vi "TestItemsIndex.vi"(6 "TestItemIndexIn":i32, 8 "ErrorIn":errorcluster, 9 "GuiRef":T1, 11 "Fail项目":string[](array[string])) -> (0 "ErrorOut":errorcluster, 1 "GuiRefOut":T1)   [LabVIEW 2013]
uses:
  GlobValue.vi
panel:
  out "Item Names":string[][](array[string])
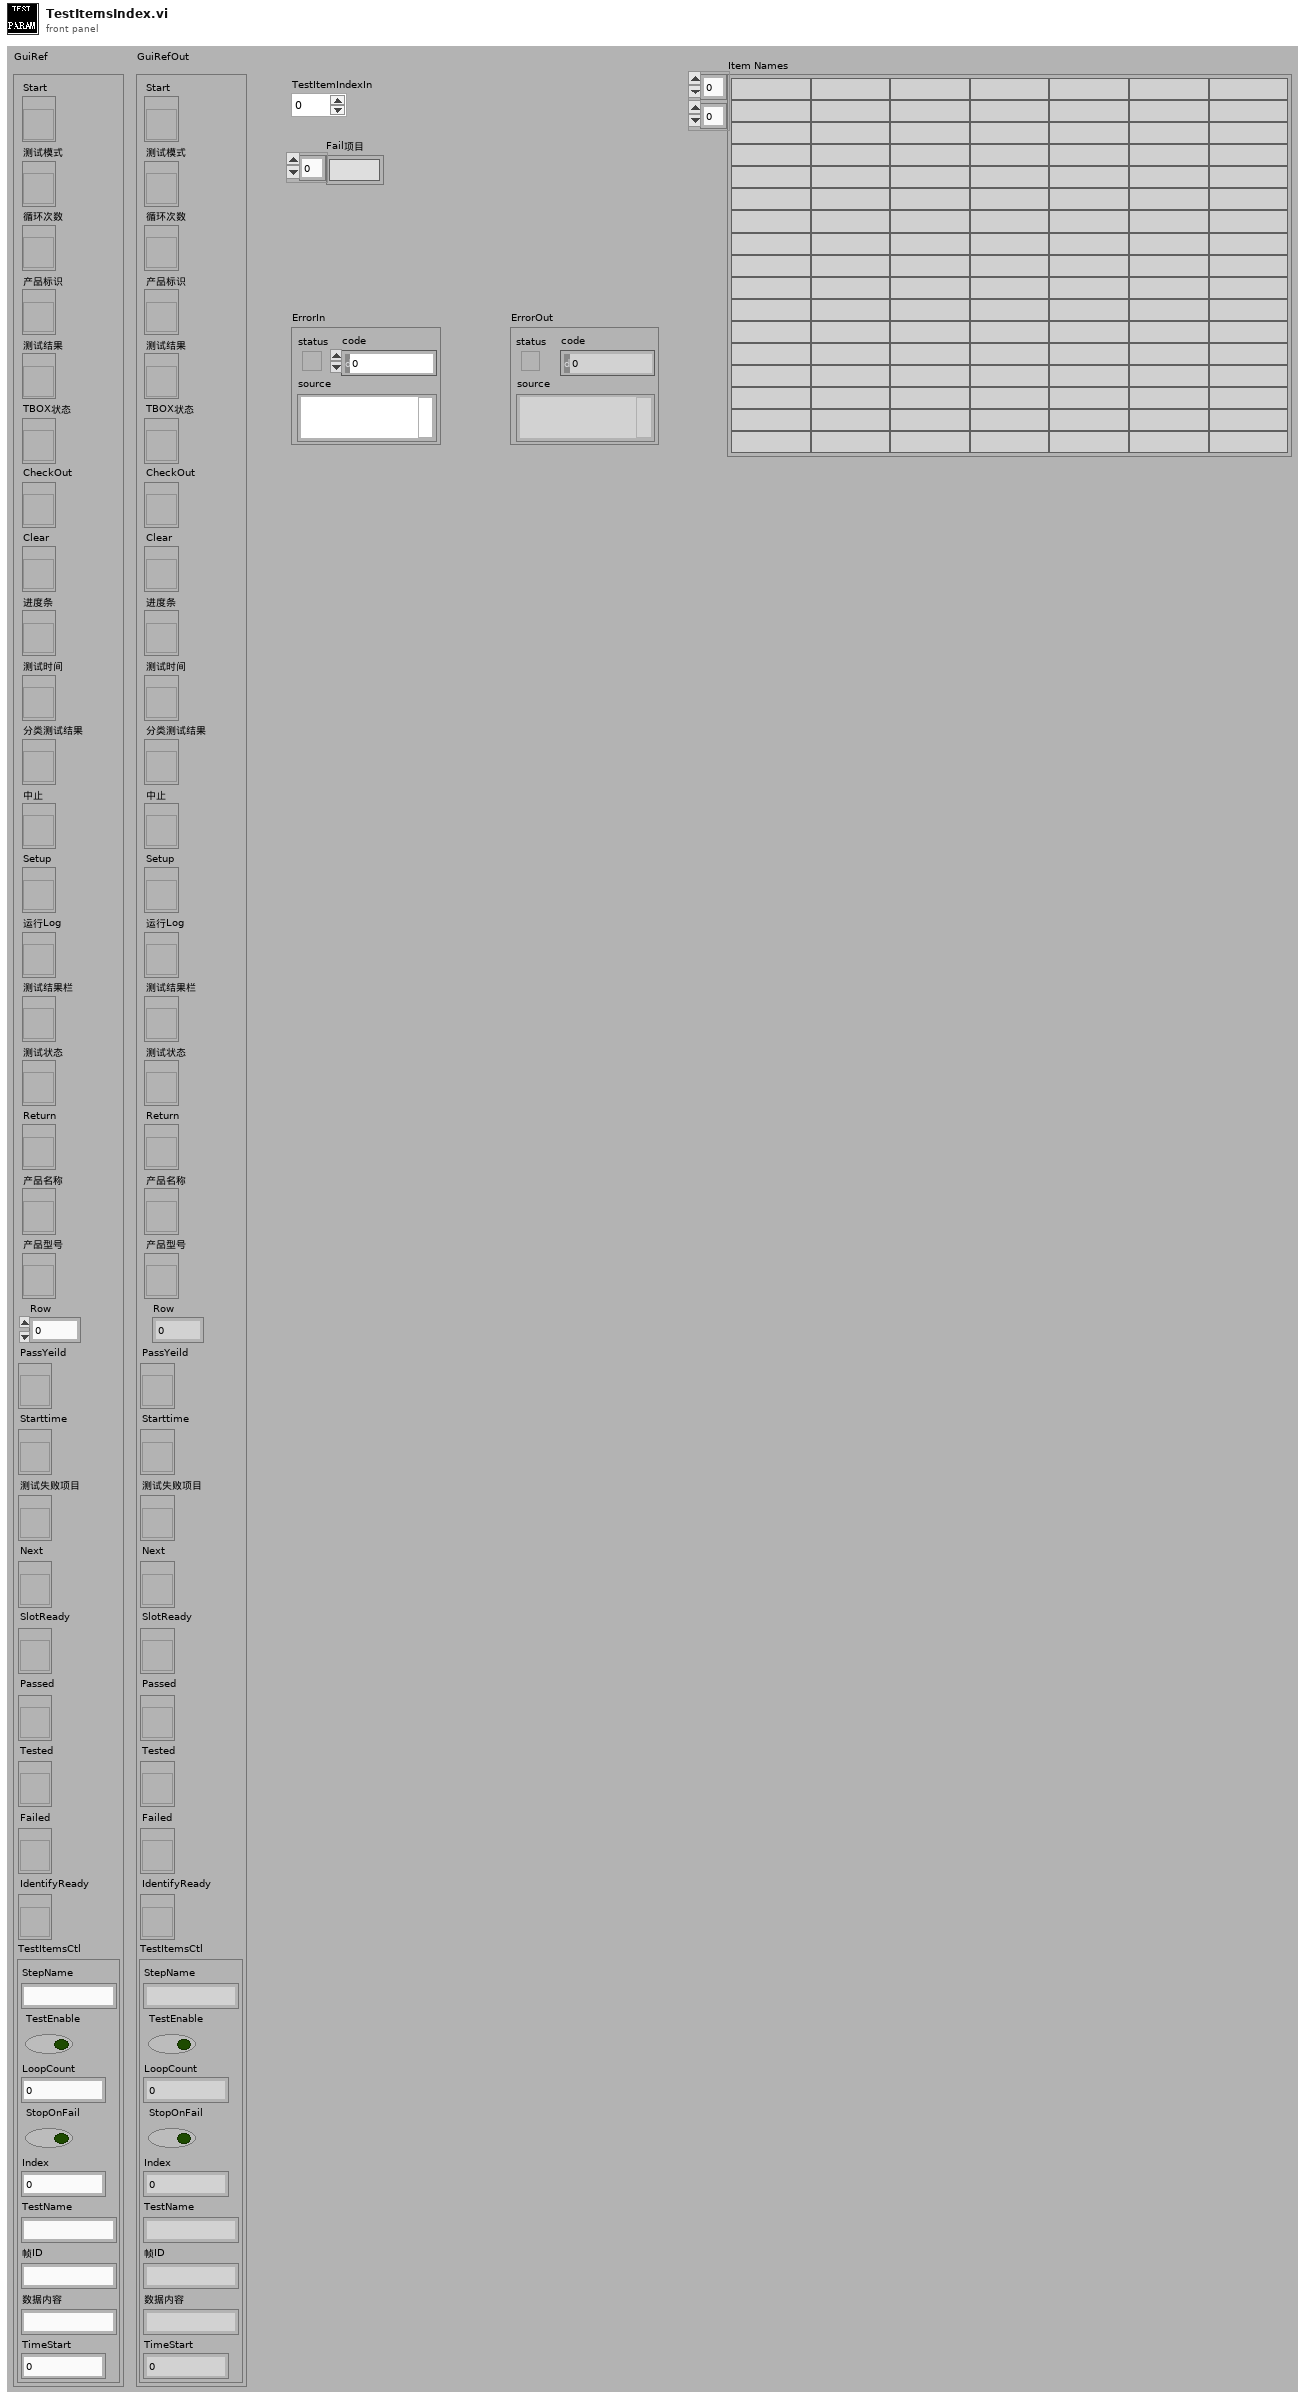
[diagram p1: front panel]
types:
  T1 = typedef "控件.ctl" = cluster{"Start":refnum<vi>, "测试模式":refnum<vi>, "循环次数":refnum<vi>, "产品标识":refnum<vi>, "测试结果":refnum<vi>, "TBOX状态":refnum<vi>, "CheckOut":refnum<vi>, "Clear":refnum<vi>, "进度条":refnum<vi>, "测试时间":refnum<vi>, "分类测试结果":refnum<vi>, "中止":refnum<vi>, "Setup":refnum<vi>, "运行Log":refnum<vi>, "测试结果栏":refnum<vi>, "测试状态":refnum<vi>, "Return":refnum<vi>, "产品名称":refnum<vi>, "产品型号":refnum<vi>, "Row":i32, "PassYeild":refnum<vi>, "Starttime":refnum<vi>, "测试失败项目":refnum<vi>, "Next":refnum<vi>, "SlotReady":refnum<vi>, "Passed":refnum<vi>, "Tested":refnum<vi>, "Failed":refnum<vi>, "IdentifyReady":refnum<vi>, "TestItemsCtl":cluster{"StepName":string, "TestEnable":bool, "LoopCount":u32, "StopOnFail":bool, "Index":u32, "TestName":string, "帧ID":string, "数据内容":string, "TimeStart":u32}}
  T2 = cluster{"StepName":string, "TestEnable":bool, "LoopCount":u32, "StopOnFail":bool, "Index":u32, "TestName":string, "帧ID":string, "数据内容":string, "TimeStart":u32}
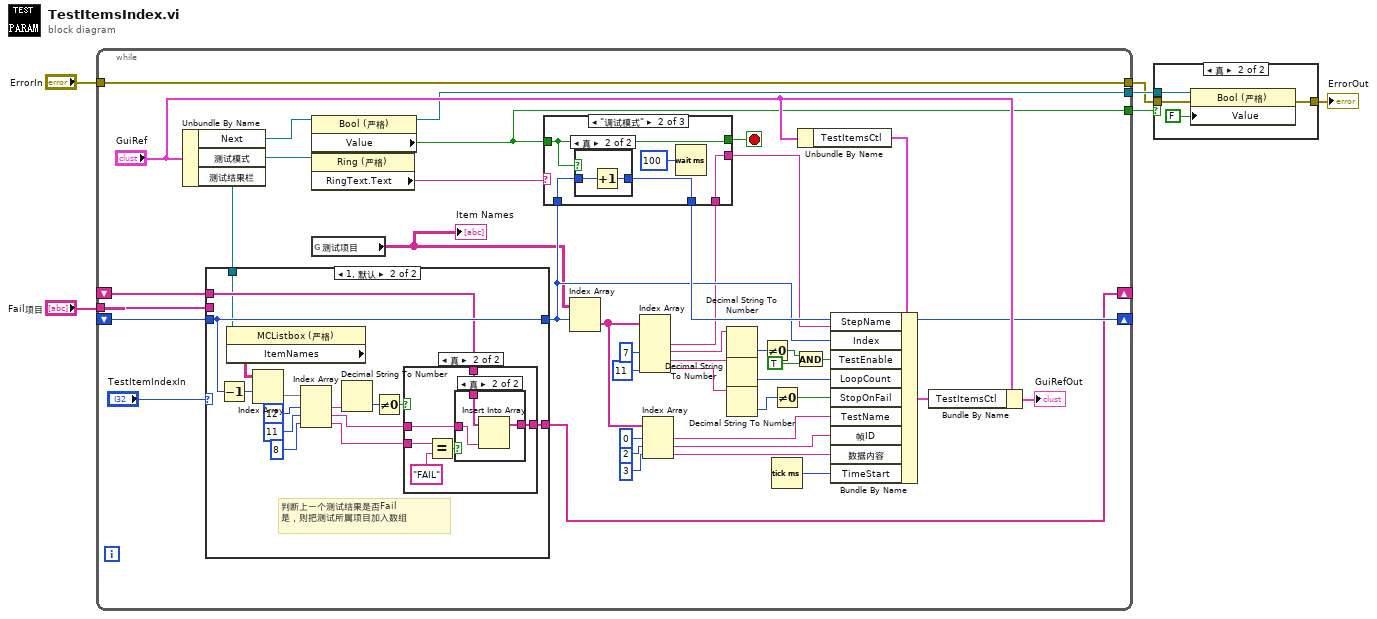
[diagram p0: block diagram]
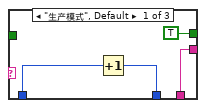
[diagram p6: hidden frame]
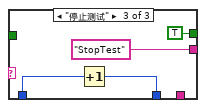
[diagram p8: hidden frame]
diagram:
  n1 = while {
    tunnel: "ErrorIn" -> [w7]
    tunnel: [w7] -> w4
    shift-right: [w30] -> _
    shift-left: _ -> [w15]
    tunnel: [w29] -> w5
    tunnel: [w28] -> w3
    shift-right: [w22] -> _
    shift-left: _ -> [w18]
    tunnel: "Fail项目" -> [w19]
    stop <- w11 stop-if-true
    n2 = Unbundle By Name("GuiRef") -> ("Next"=w33:refnum<vi>, "测试模式"=w32:refnum<vi>, "测试结果栏"=w17:refnum<vi>)
    n3 = case shown="1, 默认" "TestItemIndexIn" {
      selector: "TestItemIndexIn" -> [w50 _]
      tunnel: [w50 w63] -> w23
      tunnel: w15 -> [_ w63]
      tunnel: [w49 w62] -> w22
      tunnel: w19 -> [w49 _]
      tunnel: w18 -> [_ w61]
      tunnel: w17 -> [_ w60]
      frame 0 {
      }
      frame 1, Default {
        # "判断上一个测试结果是否Fail\n是，则把测试所属项目加入数组"
        n4 = Decrement(x=w63) -> (x-1=w65:i32)
        n5 = property class="MCListbox (严格)"(reference=w60) -> ("ItemNames"=w59:string[][])  [unwired: 1 in, 2 out]
        n6 = Index Array(array=w59, index (row)=w65) -> (element=w64:string[])  [unwired: 1 in]
        n7 = Index Array(array=w64, index #1=12 ("索引"), index #2=11 ("索引"), index #3=8 ("索引")) -> (element #1=w52:string, element #2=w55:string, element #3=w54:string)
        n8 = Decimal String To Number(string=w52) -> (number=w53:i32)  [unwired: 3 out]
        n9 = Not Equal To 0?(x=w53) -> (x != 0?=w51:bool)
        n10 = case shown="真" w51 {
          tunnel: [w66 w70] -> w62
          tunnel: w61 -> [w66 w69]
          tunnel: w55 -> [_ w68]
          tunnel: w54 -> [_ w67]
          frame False {
          }
          frame True {
            n11 = Equal?(x=w67, y="FAIL") -> (x = y?=w72:bool)
            n12 = case shown="真" w72 {
              tunnel: w68 -> [_ w76]
              tunnel: [w73 w75] -> w70
              tunnel: w69 -> [w73 w74]
              frame False {
              }
              frame True {
                n13 = Insert Into Array(array=w74, new element=w76) -> (w75:string[])  [unwired: 1 in]
              }
            }
          }
        }
      }
    }
    n14 = property class="Bool (严格)"(reference=w33) -> (reference out=w29:refnum<vi>, "Value"=w28:bool)  [unwired: 1 in, 1 out]
    n15 = property class="Ring (严格)"(reference=w32) -> ("RingText.Text"=w31:string)  [unwired: 1 in, 2 out]
    n16 = global read "GlobValue.vi" "测试项目"() -> (w16:string[][])
    "Item Names" <- w16
    n17 = Index Array(array=w16, index (row)=w23) -> (element=w44:string[])  [unwired: 1 in]
    n18 = Index Array(array=w44, index #3=7 ("index"), index #5=11 ("索引")) -> (element #2=w13:string, element #3=w41:string, element #4=w40:string, element #5=w39:string)  [unwired: 3 in, 1 out]
    n19 = case shown="\"调试模式\"" w31 {
      tunnel: w28 -> [_ w82 _]
      tunnel: w23 -> [w80 w85 w92]
      tunnel: [w79 w84 w91] -> w30
      tunnel: [TRUE w82 TRUE] -> w11
      tunnel: w13 -> [w78 w81 _]
      tunnel: [w78 w81 "StopTest" ("element")] -> w12
      frame "生产模式", Default {
        n20 = Increment(x=w80) -> (x+1=w79:i32)
      }
      frame "调试模式" {
        n21 = case shown="真" w82 {
          tunnel: w85 -> [w86 w88]
          tunnel: [w86 w87] -> w84
          frame False {
          }
          frame True {
            n22 = Increment(x=w88) -> (x+1=w87:i32)
          }
        }
        n23 = Wait (ms)(milliseconds to wait=u32 100) -> ()  [unwired: 1 out]
      }
      frame "停止测试" {
        n24 = Increment(x=w92) -> (x+1=w91:i32)
      }
    }
    n25 = Index Array(array=w44, index #1=0 ("索引"), index #2=2 ("索引"), index #3=3 ("索引")) -> (element #1=w10:string, element #2=w43:string, element #3=w42:string)
    n26 = Decimal String To Number(string=w41) -> (number=w48:i32)  [unwired: 3 out]
    n27 = Decimal String To Number(string=w40) -> (number=w45:i32)  [unwired: 3 out]
    n28 = Decimal String To Number(string=w39) -> (number=w47:i32)  [unwired: 3 out]
    n29 = Not Equal To 0?(x=w48) -> (x != 0?=w21:bool)
    n30 = Not Equal To 0?(x=w47) -> (x != 0?=w46:bool)
    n31 = Tick Count (ms)() -> (millisecond timer value=w24:u32)
    n32 = And(x=w21, y=TRUE) -> (x .and. y?=w20:bool)
    n33 = Unbundle By Name("GuiRef") -> ("TestItemsCtl"=w35:T2)
    n34 = Bundle By Name(cluster=w35, "StepName"=w12, "Index"=w23, "TestEnable"=w20, "LoopCount"=w45, "StopOnFail"=w46, "TestName"=w10, "帧ID"=w43, "数据内容"=w42, "TimeStart"=w24) -> (w37:T2)
    n35 = Bundle By Name(cluster="GuiRef", "TestItemsCtl"=w37) -> (→"GuiRefOut":T1)
  }
  n36 = case shown="真" w3 {
    tunnel: w5 -> [_ w97]
    tunnel: w4 -> [w93 w95]
    tunnel: [w93 w94] -> w1
    frame False {
    }
    frame True {
      n37 = property class="Bool (严格)"(reference=w97, error in=w95, "Value"=FALSE) -> (error out=w94:errorcluster)  [unwired: 1 out]
    }
  }
  "ErrorOut" <- w1
